vi "SteerGlobals.vi"() -> ()   [LabVIEW 2014]
panel:
  in  "SteerFR":dbl
  in  "SteerFL":dbl
  in  "SteerBR":dbl
  in  "SteerBL":dbl
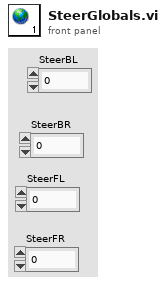
[diagram p1: front panel]
diagram:
